vi "to string.vi"(8 "error in":errorcluster, 11 "Modbus Slave configuration in":refnum<class "Modbus Module configuration.lvclass">) -> (0 "error out":errorcluster, 1 "data":string, 2 "version":string, 3 "Modbus Slave configuration out":refnum<class "Modbus Module configuration.lvclass">)   [LabVIEW 2013, in "Modbus Module configuration.lvclass"]
doc: "Provides an interface for saving a module configuration to a file or other serialized data source. It is recommended that all children of this class store data in two sets--data required for its own initialization, and any data required for parent initialization--and that each implementation uses the <b>Call Parent Method</b> primitive to serialize parent information.Platypus Framework 1.0.1.65\nNI Systems Engineering - National Instruments"
uses:
  Modbus Module configuration.lvclass
  <vilib>/NI/Tag Bus Module Framework/module configuration/TBM module configuration.lvclass
  Modbus Module configuration.lvclass/Modbus Module configuration.ctl
  module channel/Modbus Module Channel.lvclass
  <vilib>/NI/Configuration Framework/serializable configuration/NISE_CEF_serializable configuration.lvclass
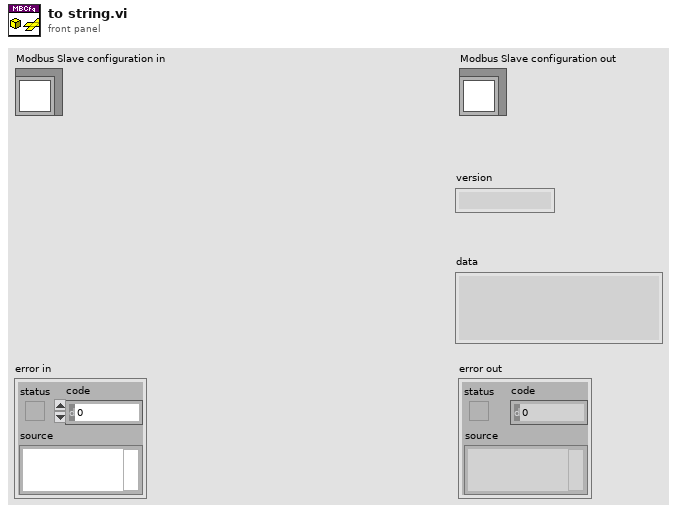
[diagram p1: front panel]
types:
  T1 = typedef "Modbus Module configuration.lvclass/modbus class.ctl" = enum16{"TCP master", "TCP slave", "serial master", "serial slave"}
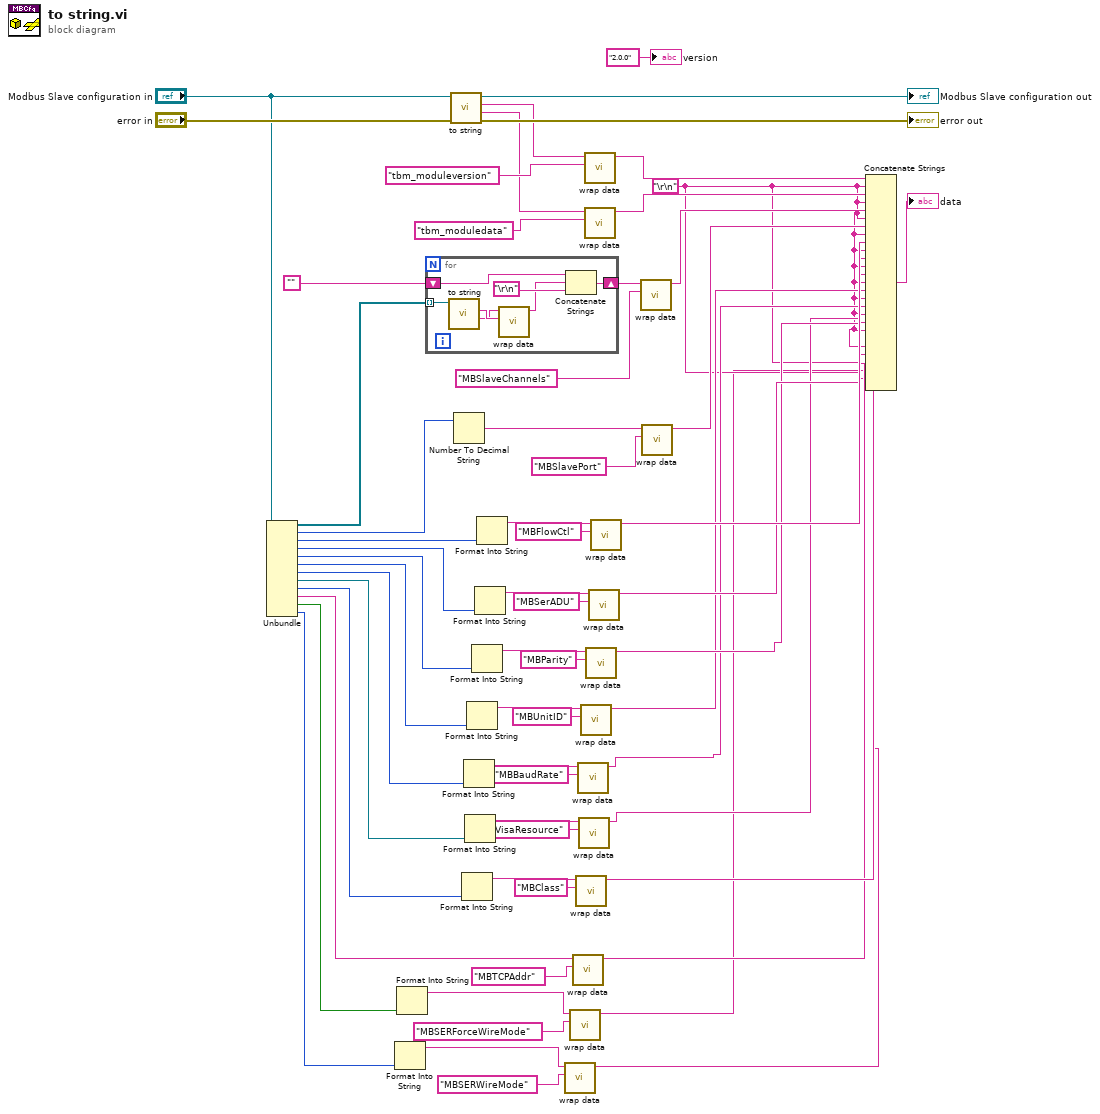
[diagram p0: block diagram]
diagram:
  w3 = "\r\n"
  n1 = Unbundle("Modbus Slave configuration in") -> (w48:refnum<class "Modbus Module Channel.lvclass">[], w43:u16, w39:u16, w25:enum16{"RTU", "ASCII"}, w24:u16, w23:u8, w22:u32, w21:refnum<visa-resource-name>, w20:T1, w12:string, w6:bool, w7:i16)
  n2 = Format Into String(w7) -> (resulting string=w4:string)  [unwired: 3 in, 1 out]
  n3 = Format Into String(w6) -> (resulting string=w5:string)  [unwired: 3 in, 1 out]
  n4 = for {
    tunnel: w48 -> [w64] mode=indexing
    shift-right: [w67] -> w46
    shift-left: "" -> [w66]
    n5 = call-dynamic "to string.vi"("channel in"=w64) -> ("channel data"=w62:string, "identifier"=w63:string)  [unwired: 7 in, 2 out]
    n6 = call <vilib>:"wrap data.vi"("identifier"=w63, "data to wrap"=w62) -> ("wrapped data"=w65:string)  [unwired: 9 in]
    n7 = Concatenate Strings(w66, w65, "\r\n") -> (w67:string)
  }
  n8 = call-parent "to string.vi"("error in"="error in", "module configuration in"="Modbus Slave configuration in") -> ("error out"=→"error out":errorcluster, "data"=w53:string, "version"=w54:string, "module configuration out"=→"Modbus Slave configuration out":refnum<class "Modbus Module configuration.lvclass">)  [unwired: 6 in]
  n9 = Number To Decimal String(number=w43) -> (decimal integer string=w42:string)  [unwired: 1 in]
  n10 = Format Into String(w20) -> (resulting string=w27:string)  [unwired: 3 in, 1 out]
  n11 = Format Into String(w22) -> (resulting string=w32:string)  [unwired: 3 in, 1 out]
  n12 = Format Into String(w21) -> (resulting string=w28:string)  [unwired: 3 in, 1 out]
  n13 = Format Into String(w23) -> (resulting string=w31:string)  [unwired: 3 in, 1 out]
  n14 = Format Into String(w24) -> (resulting string=w35:string)  [unwired: 3 in, 1 out]
  n15 = Format Into String(w25) -> (resulting string=w36:string)  [unwired: 3 in, 1 out]
  n16 = Format Into String(w39) -> (resulting string=w40:string)  [unwired: 3 in, 1 out]
  n17 = call <vilib>:"wrap data.vi"("identifier"="MBSERWireMode", "data to wrap"=w4) -> ("wrapped data"=w1:string)  [unwired: 9 in]
  n18 = call <vilib>:"wrap data.vi"("identifier"="MBSERForceWireMode", "data to wrap"=w5) -> ("wrapped data"=w2:string)  [unwired: 9 in]
  n19 = call <vilib>:"wrap data.vi"("identifier"="MBTCPAddr", "data to wrap"=w12) -> ("wrapped data"=w11:string)  [unwired: 9 in]
  n20 = call <vilib>:"wrap data.vi"("identifier"="MBClass", "data to wrap"=w27) -> ("wrapped data"=w13:string)  [unwired: 9 in]
  n21 = call <vilib>:"wrap data.vi"("identifier"="MBBaudRate", "data to wrap"=w32) -> ("wrapped data"=w15:string)  [unwired: 9 in]
  n22 = call <vilib>:"wrap data.vi"("identifier"="MBVisaResource", "data to wrap"=w28) -> ("wrapped data"=w14:string)  [unwired: 9 in]
  n23 = call <vilib>:"wrap data.vi"("identifier"="MBUnitID", "data to wrap"=w31) -> ("wrapped data"=w16:string)  [unwired: 9 in]
  n24 = call <vilib>:"wrap data.vi"("identifier"="tbm_moduleversion" ("additional identifier"), "data to wrap"=w54) -> ("wrapped data"=w56:string)  [unwired: 9 in]
  n25 = call <vilib>:"wrap data.vi"("identifier"="tbm_moduledata" ("additional identifier"), "data to wrap"=w53) -> ("wrapped data"=w55:string)  [unwired: 9 in]
  n26 = call <vilib>:"wrap data.vi"("identifier"="MBParity", "data to wrap"=w35) -> ("wrapped data"=w17:string)  [unwired: 9 in]
  n27 = call <vilib>:"wrap data.vi"("identifier"="MBSerADU", "data to wrap"=w36) -> ("wrapped data"=w18:string)  [unwired: 9 in]
  n28 = call <vilib>:"wrap data.vi"("identifier"="MBFlowCtl", "data to wrap"=w40) -> ("wrapped data"=w19:string)  [unwired: 9 in]
  n29 = call <vilib>:"wrap data.vi"("identifier"="MBSlaveChannels" ("additional identifier"), "data to wrap"=w46) -> ("wrapped data"=w50:string)  [unwired: 9 in]
  n30 = call <vilib>:"wrap data.vi"("identifier"="MBSlavePort" ("additional identifier"), "data to wrap"=w42) -> ("wrapped data"=w44:string)  [unwired: 9 in]
  n31 = Concatenate Strings(w56, w3, w55, w3, w50, w3, w44, w3, w19, w3, w18, w3, w17, w3, w16, w3, w15, w3, w14, w3, w13, w3, w11, w3, w2, w3, w1) -> (→"data":string)
  "version" <- "2.0.0" ("current version")
